vi "NI 5772 (AC) - Digitizer_vDirectDataSend (FPGA) Averaging Try1.vi"() -> ()   [LabVIEW 2020]
doc: "Example Description:\nThis example demonstrates how to enable Time Interleaved Sampling with the NI 5772 adapter module to achieve a sampling rate of 1.6GS/s. This example continuously acquires records of analog input data from the NI 5772 adapter module. It allows you to select an AI channel, trigger type, and record size. This VI must be compiled before it is run. \n\nRunning the VI:\nThis VI must be run from the NI 5772 - Getting Started (Host).vi. Refer to the host VI documentation for steps regarding running and configuring the FPGA VI. \n\nExecution Steps:\nRefer to the Block Diagram of this VI for execution comments."
uses:
  Controls/AI Trigger Type.ctl
  Controls/Aquire State.ctl
  <vilib>/Platform/TimedLoop/XDataNode/timing_clust.ctl
  <vilib>/Platform/TimedLoop/XDataNode/nitl_modes.ctl
  <vilib>/Platform/TimedLoop/XDataNode/wakeup.ctl
  Controls/DigitizerState.ctl
  <vilib>/rvi/Emulation/niFpgaGetClockAttributes.vi
  <vilib>/rvi/Emulation/niFpgaSctlEmulationGetInTimedLoop.vi
  <vilib>/rvi/Emulation/niFpgaEmulationReportErrorSimple.vi
  <vilib>/rvi/eio/common/nirviEmuTemplateMethod_errors.vi
  <vilib>/rvi/Emulation/niFpgaCriticalErrorInLSC.vi
  <vilib>/rvi/Emulation/niFpgaProcessEmulError.vi
  <vilib>/rvi/Emulation/niFpgaEmulationIsFPGAContextNoSignature.vi
  <vilib>/rvi/errors/niFpgaSetErrorForExecOnDevCompSimple.vi
  <vilib>/rvi/eio/common/nirviEmuReportErrorAndStop.vi
  <vilib>/rvi/DataTransferAndStorage/Container/Common/niFpgaContainerGetUniqueNameForEmu.vi
  <vilib>/rvi/FIFO/Fifo_Resource/nirvififoEmulationSetSize.vi
  <vilib>/rvi/FIFO/Fifo_Resource/nirviFifoEmulationQueueMgr.vi
  <instcachedir>/0/nirviFifoEmulationQueueMgr_E5CAEC123FF24DC58D834DCA3CDAA9B5.lvgen/nirviFifoEmulationQueueMgr_E5CAEC123FF24DC58D834DCA3CDAA9B5_004.vi
  <vilib>/Utility/error.llb/Clear Errors.vi
  <vilib>/rvi/FIFO/Fifo_Resource/nirvififoEmulationCreateLock.vi
  <vilib>/rvi/FIFO/Fifo_Resource/nirvififoEmulationObtainLock.vi
  <vilib>/rvi/FIFO/Fifo_Resource/nirvififoEmulationReleaseLock.vi
  <vilib>/rvi/occurrence/nirviWaitOnOccurrenceBase.vi
  <vilib>/rvi/errors/nirviReportUnexpectedCaseInternalError.vi
  <vilib>/rvi/errors/nirviReportUnexpectedCaseInternalError (U32).vi
  <instcachedir>/0/nirviFifoEmulationQueueMgr_E5CAEC123FF24DC58D834DCA3CDAA9B5.lvgen/nirviFifoEmulationQueueMgr_E5CAEC123FF24DC58D834DCA3CDAA9B5_009.vi
  <vilib>/rvi/FIFO/Fifo_Resource/nirvififoEmulationDetermineInputValidOut.vi
  <instcachedir>/0/nirviFifoEmulationQueueMgr_E5CAEC123FF24DC58D834DCA3CDAA9B5.lvgen/nirviFifoEmulationQueueMgr_E5CAEC123FF24DC58D834DCA3CDAA9B5_000.vi
  <vilib>/rvi/interface/RandomDataEmulation/niFpgaRandomDataHandleErrors.vi
  <instrlib>/_niInstr/Basic Elements/v1/FPGA/Private/Count Up U64.vi
  <vilib>/eio/EIONode/EIONode.xnode
  <vilib>/rvi/DataTransferAndStorage/Container/XNode/niFpgaContainer.xnode
  <vilib>/rvi/FIFO/Fifo_Resource/nirvififoEmulationRead.vi
  <vilib>/Platform/TimedLoop/XDataNode/XDataNode.xnode
  <vilib>/rvi/FIFO/Fifo_Resource/nirvififoEmulationGetNumberOfElementsToRead.vi
  <vilib>/rvi/FIFO/Fifo_Resource/nirvififoEmulationWrite.vi
  <vilib>/rvi/interface/RandomDataEmulation/nirviRandomDataFpgaReadWriteTemplate.vi
  <vilib>/Platform/TimedLoop/XDataNode/XDNodeRunTimeDep.lvlib
  <instrlib>/_niInstr/Basic Elements/v1/FPGA/niInstr Basic Elements v1 FPGA.lvlib
  <vilib>/rvi/Memory/Memory_Emulation/nirvimemoryFastEmulation.vi
  <vilib>/rvi/Memory/Memory_Emulation/nirvimemoryEmulation.vi
panel:
  out "DMA FIFO Overflow? 3":bool caption="FIFO Overflow?"
  out "DMA FIFO Overflow? 2":bool caption="FIFO Overflow?"
  out "WaitForWave\nCompletion":u16
  in  "Wave Sampling Rate":sgl
  in  "WaveSampleCount":sgl format="%#_13g"
  in  "Delay (us)":sgl
  in  "AvgCount_powerOf2":i16=1
  out "DMA FIFO Overflow?":bool caption="FIFO Overflow?"
  out "Removed\nElement":u64
  out "AvgCount":u16=1
  in  "vi/nGenTrig":bool
  in  "TrigIn Simulate":bool
  out "Trig Count":u64
  in  "Clear Count":bool
  out "Delay after Trig [cycles]":u16
  out "TS FIFO In Overflow?":bool caption="FIFO Overflow?"
  in  "Samples Per Trigger":u16=512 min=1 step=1
  in  "Arm Trigger":bool
  in  "User Command Commit":bool
  in  "User Command":u8
  out "User Command Idle":bool
  out "User Command Status":u8
  in  "User Data 0":u16
  in  "User Data 1":u8
  out "PLL Locked":bool
  out "User Error":bool
  out "Configured?":bool
  in  "Trigger Level":i16
  in  "Trigger Type":T1
  # "Resource Configuration"
  # "Analog Input"
  # "Clock Configuration"
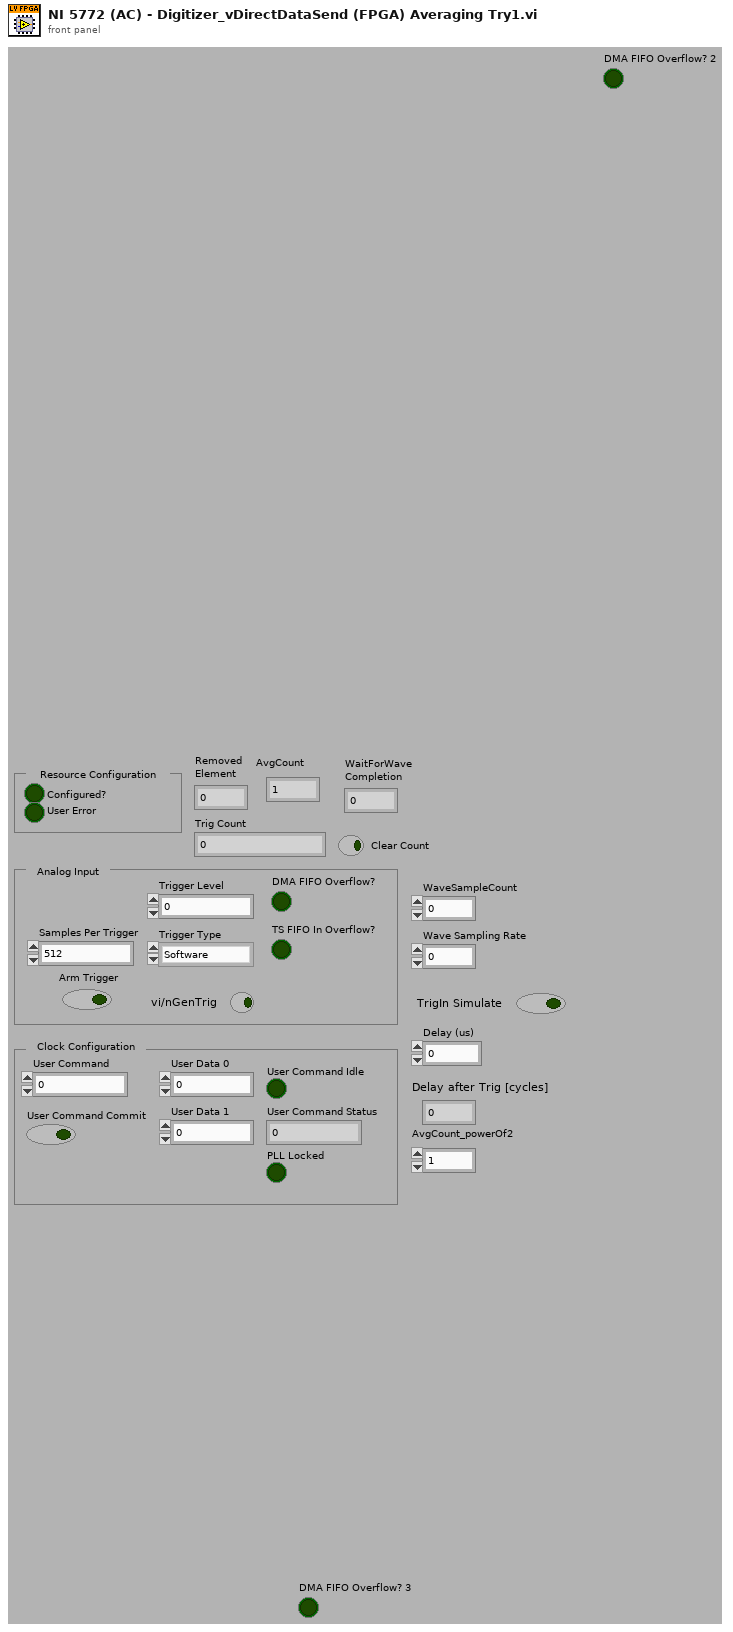
[diagram p1: front panel]
types:
  T1 = typedef "AI Trigger Type.ctl" = enum8{"Software", "Data Edge"}
  T2 = typedef "DigitizerState.ctl" = enum16{"Init", "Build/Clear Accumulator", "GetData", "AverageCountCheck", "SendtoHost"}
  T3 = typedef "Aquire State.ctl" = enum8{"Idle", "Wait for Trigger", "AlignWave", "Hold Aquire", "Acquire", "WaitForWaveCompletion", "CheckAvg"}
  T4 = typedef "XDNodeRunTimeDep.lvlib/timing_clust.ctl" = cluster{"Expected End [f-1]":u64, "Actual End [f-1]":u64, "Finished Late? [f-1]":bool, "Expected End [i-1]":u64, "Actual End [i-1]":u64, "Finished Late? [i-1]":bool, "Expected Start [i]":u64, "Actual Start [i]":u64, "Expected Start [f]":u64, "Actual Start [f]":u64, "Source Name":string, "Structure Name":string, "Period":i64, "Deadline":i64, "Offset":i64, "Start":i64, "Priority":i32, "Timeout":i32, "Mode":T5, "Wakeup Reason":T6, "Error":errorcluster, "Source Type":string, "Secondary Source Type":string, "Global End Time":u64, "Global Start Time":u64, "Frame Duration":u64, "Iteration Duration":u64, "Assigned CPU":i32, "I/O Scan Engine Mode":u32}
  T5 = typedef "XDNodeRunTimeDep.lvlib/nitl_modes.ctl" = enum32{"No Change", "Process missed periods, maintain original phase", "Discard missed periods, maintain original phase", "Process missed periods, ignore original phase", "Discard missed periods, ignore original phase"}
  T6 = typedef "XDNodeRunTimeDep.lvlib/wakeup.ctl" = enum32{"Normal", "Aborted", "Asynchronous wakeup", "Timing source error", "Timed loop error", "Timeout"}
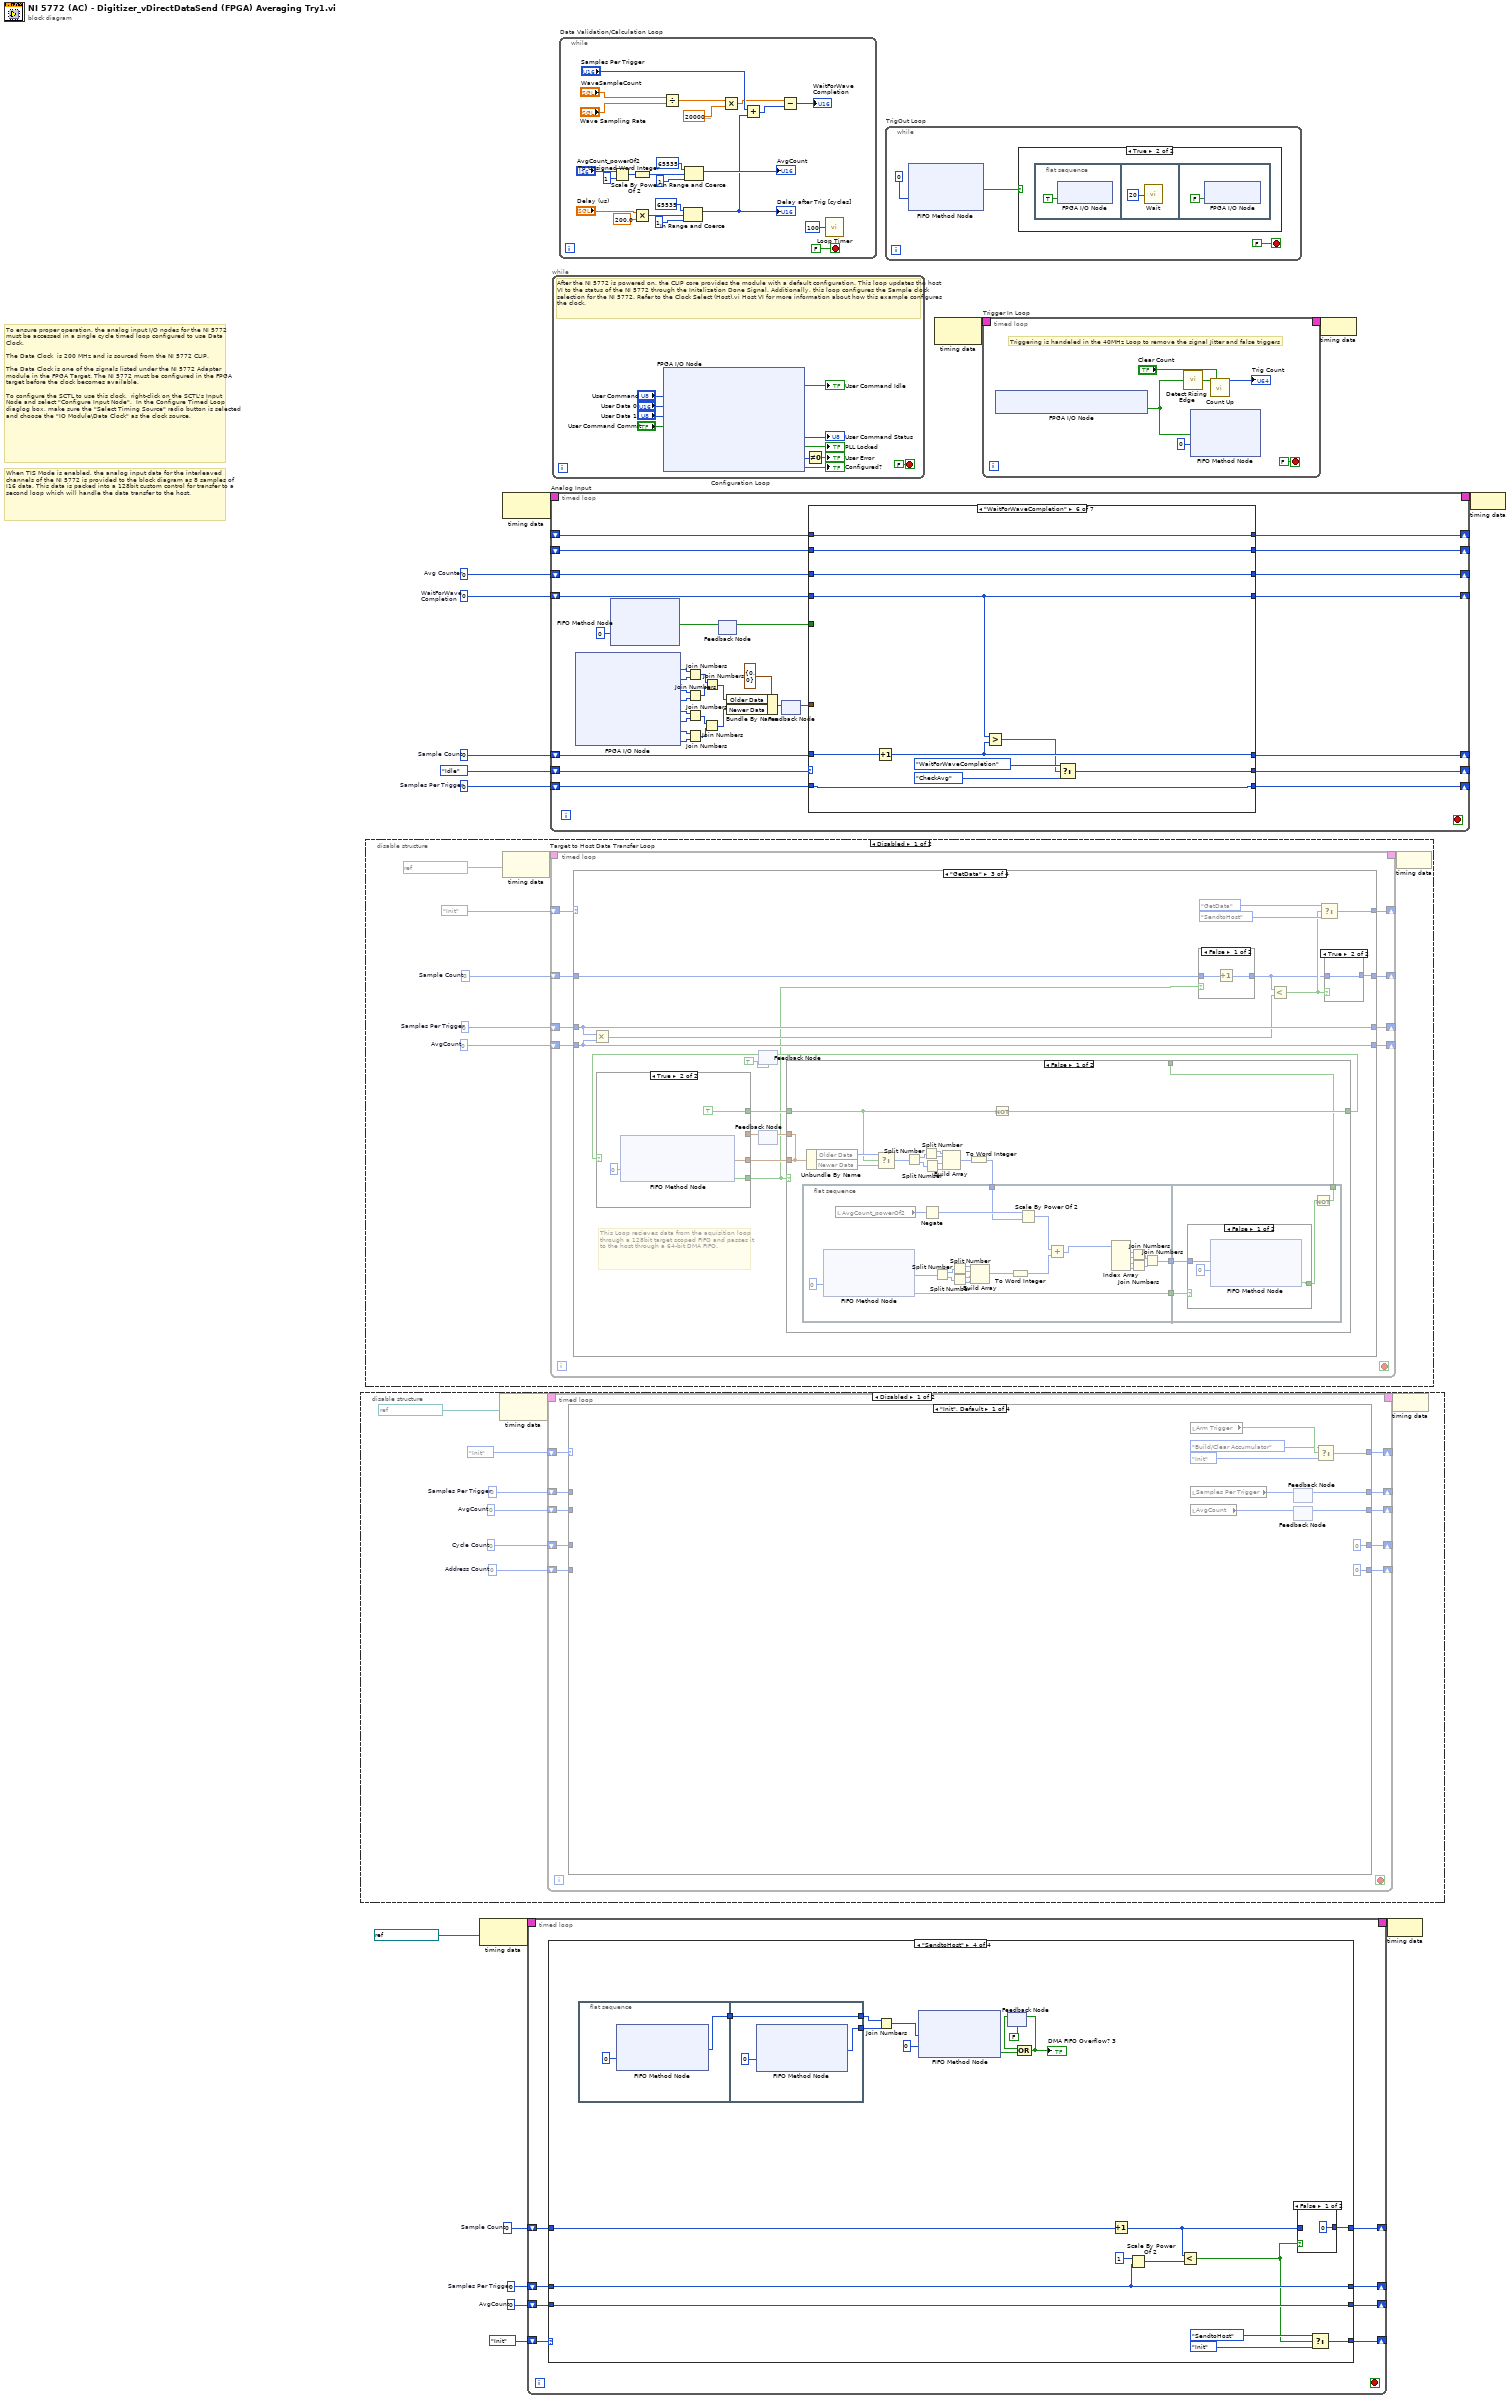
[diagram p0: block diagram]
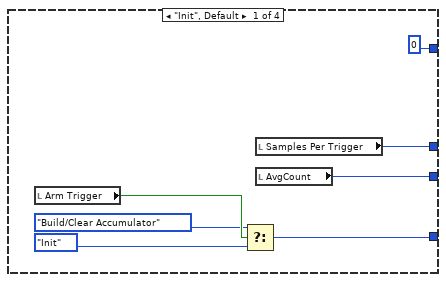
[diagram p2: hidden frame]
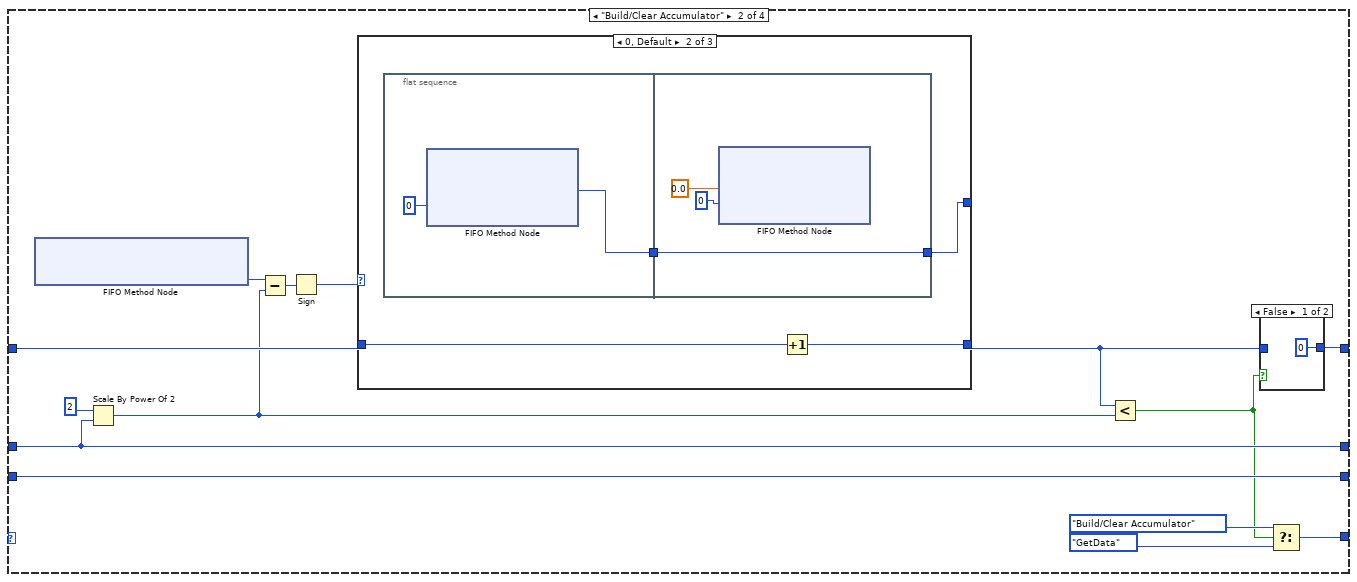
[diagram p3: hidden frame]
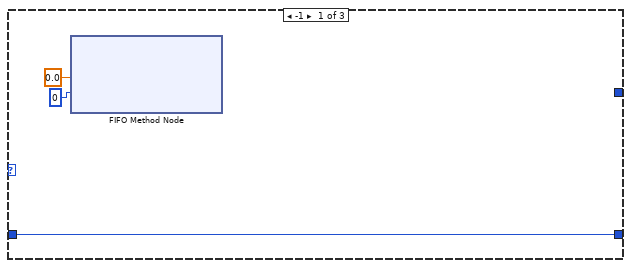
[diagram p5: hidden frame]
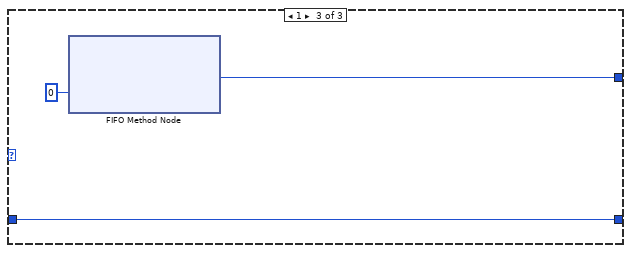
[diagram p6: hidden frame]
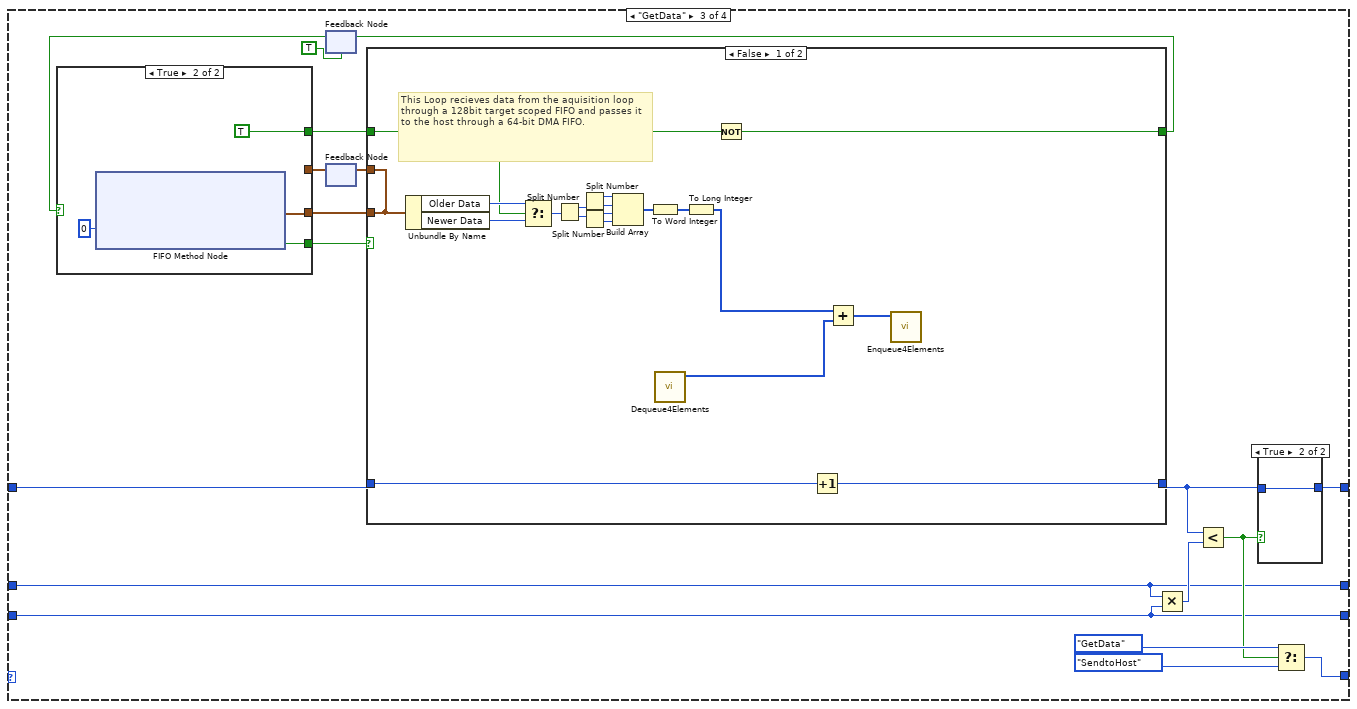
[diagram p7: hidden frame]
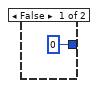
[diagram p8: hidden frame]
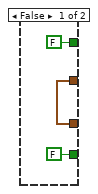
[diagram p9: hidden frame]
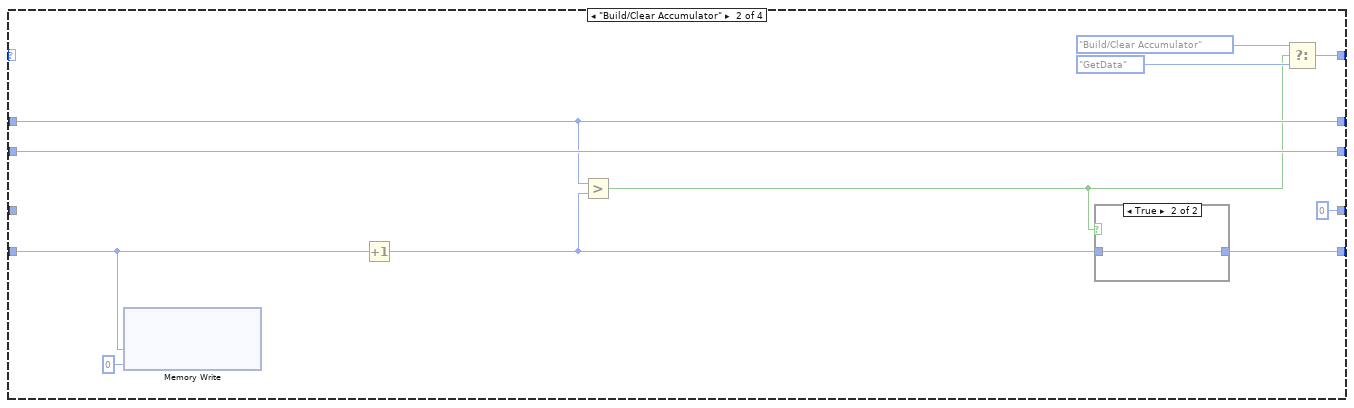
[diagram p12: hidden frame]
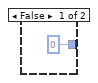
[diagram p13: hidden frame]
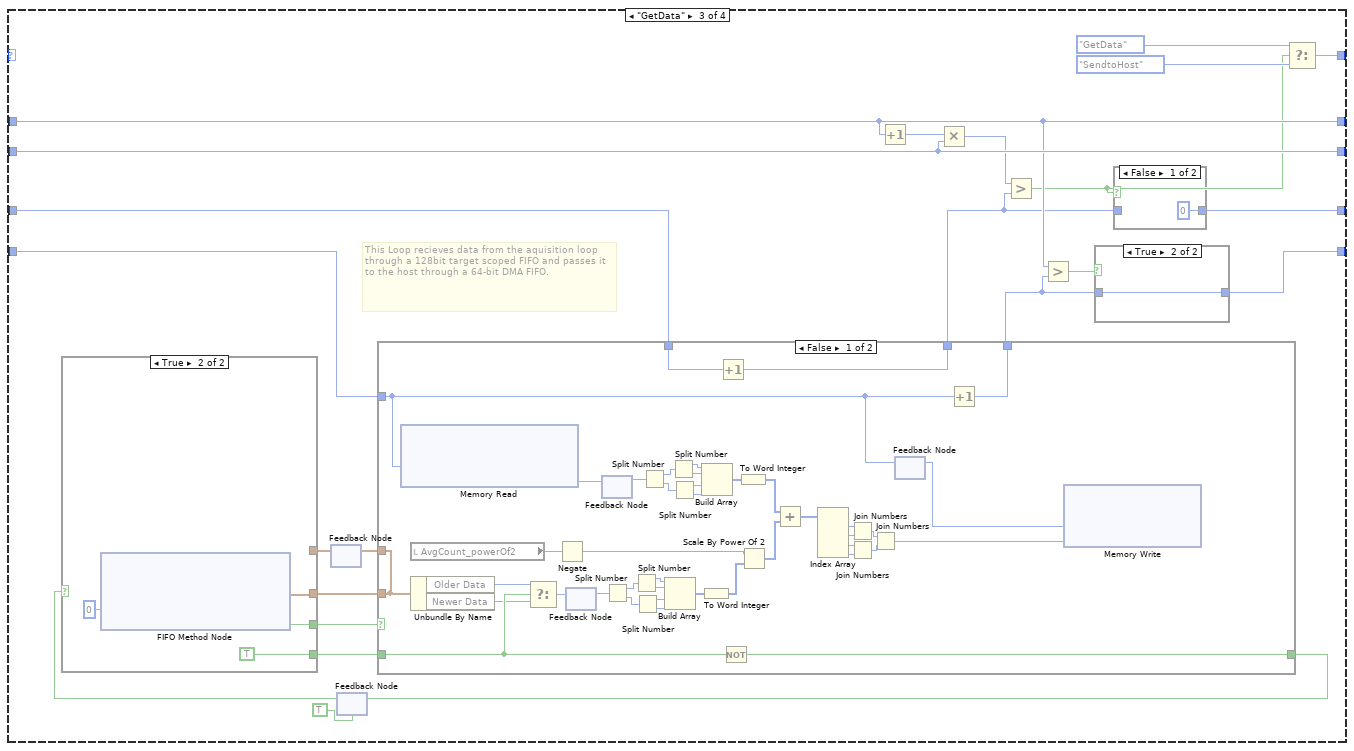
[diagram p14: hidden frame]
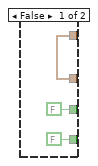
[diagram p16: hidden frame]
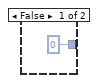
[diagram p18: hidden frame]
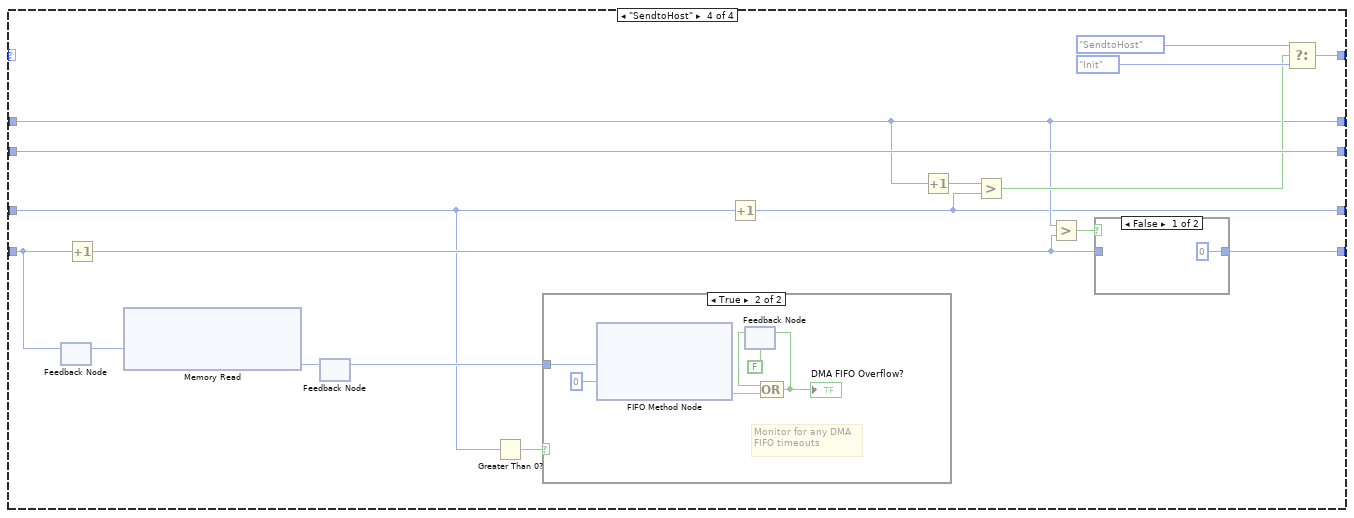
[diagram p19: hidden frame]
diagram:
  w1 = u16 0  # Sample Count
  w2 = u16 0  # AvgCount
  w3 = u16 0  # Samples Per Trigger
  w8 = u16 0  # WaitForWave Completion
  w9 = u16 0  # Avg Counter
  w12 = u16 0  # Samples Per Trigger
  w13 = u16 0  # Sample Count
  # "When TIS Mode is enabled, the analog input data for the interleaved channels of the NI 5772 is provided to the block diagram as 8 samples of I16 data. This data is packed into a 128bit custom control for transfer to a second loop which will handle the data transfer to the host."
  # "To ensure proper operation, the analog input I/O nodes for the NI 5772 must be accessed in a single cycle timed loop configured to use Data Clock. \n\nThe Data Clock  is 200 MHz and is sourced from the NI 5772 CLIP.\n\nThe Data Clock is one of the signals listed under the NI 5772 Adapter module in the FPGA Target. The NI 5772 must be configured in the FPGA target before the clock becomes available. \n\nTo configure the SCTL to use this clock,  right-click on the SCTL's Input Node and select \"Configure Input Node\".  In the Configure Timed Loop diaglog box, make sure the \"Select Timing Source\" radio button is selected and choose the \"IO Module\\Data Clock\" as the clock source."
  n1 = disable-structure shown="Disabled" {
    frame Disabled {
      w17 = u32 0  # Cycle Count
      w18 = u32 0  # Address Count
      w19 = u16 0  # AvgCount
      w20 = u16 0  # Samples Per Trigger
      n2 = node-c288(refnum<k21> "100 MHz Clock" ("Source Name")) -> (w24:T4)
      n3 = timed-loop {
        timing: w24 -> [_]
        timing-out: [_] -> w23
        shift-right: [w33] -> _
        shift-left: DigitizerState."Init" -> [w34]
        shift-right: [w32] -> _
        shift-left: w20 -> [w30]
        shift-right: [w31] -> _
        shift-left: w19 -> [w29]
        shift-right: [w27] -> _
        shift-left: w18 -> [w28]
        shift-right: [w25] -> _
        shift-left: w17 -> [w26]
        stop <- _ stop-if-true
        n4 = case shown="\"Init\", Default" w34 {
          tunnel: [w39 w49 w78 w150] -> w33
          tunnel: [w38 w52 w62 w140] -> w32
          tunnel: [w37 w53 w68 w153] -> w31
          tunnel: w30 -> [_ w52 w62 w140]
          tunnel: w29 -> [_ w53 w68 w153]
          tunnel: w28 -> [_ w55 w65 w142]
          tunnel: [u32 0 w46 w77 w148] -> w27
          tunnel: w26 -> [_ _ w61 w137]
          tunnel: [u32 0 ("Cycle Count") u32 0 ("Cycle Count") w58 w138] -> w25
          frame "Init", Default {
            n5 = local read "Arm Trigger"() -> (w44:bool)
            n6 = local read "Samples Per Trigger"() -> (w40:u16)
            n7 = local read "AvgCount"() -> (w41:u16)
            n8 = feedback #1() -> (w38:u16)  [unwired: 1 in]
            n9 = feedback-in #1(w40) -> ()
            n10 = feedback #2() -> (w37:u16)  [unwired: 1 in]
            n11 = feedback-in #2(w41) -> ()
            n12 = Select(t=DigitizerState."Build/Clear Accumulator", s=w44, f=DigitizerState."Init") -> (s? t:f=w39:T2)
          }
          frame "Build/Clear Accumulator" {
            n13 = xnode ("Memory Write")("Address"=w55, "Data"=u64 0) -> ()  [unwired: 1 in, 1 out]
            n14 = Increment(x=w55) -> (x+1=w47:u32)
            n15 = Greater?(x=w52, y=w47) -> (0:w48:bool)
            n16 = case shown="True" w48 {
              tunnel: w47 -> [_ w57]
              tunnel: [u32 0 w57] -> w46
              frame False {
              }
              frame True {
              }
            }
            n17 = Select(t=DigitizerState."Build/Clear Accumulator", s=w48, f=DigitizerState."GetData") -> (s? t:f=w49:T2)
          }
          frame "GetData" {
            # "This Loop recieves data from the aquisition loop through a 128bit target scoped FIFO and passes it to the host through a 64-bit DMA FIFO."
            n18 = feedback #3() -> (w72:cluster{"Older Data":u64, "Newer Data":u64})  [unwired: 1 in]
            n19 = feedback #4(TRUE ("Timed Out?")) -> (w71:bool)
            n20 = case shown="True" w71 {
              tunnel: [w83 w86] -> w74
              tunnel: [FALSE ("Timed Out?") w87] -> w76
              tunnel: [FALSE ("Timed Out?") TRUE ("Timed Out?")] -> w75
              tunnel: w72 -> [w83 _]
              frame False {
              }
              frame True {
                n21 = xnode ("FIFO Method Node")("Timeout"=0) -> ("Element"=w86:cluster{"Older Data":u64, "Newer Data":u64}, "Timed Out?"=w87:bool)  [unwired: 1 in, 1 out]
              }
            }
            n22 = case shown="False" w76 {
              tunnel: [w128 w134] -> w70
              tunnel: w75 -> [w129 w134]
              tunnel: w74 -> [w127 w133]
              tunnel: [w127 w133] -> w73
              tunnel: w65 -> [w104 w132]
              tunnel: [w117 w132] -> w64
              tunnel: w61 -> [w93 w131]
              tunnel: [w92 w131] -> w59
              frame False {
                n23 = xnode ("Memory Read")("Address"=w104) -> ("Data"=w95:u64)  [unwired: 1 in, 1 out]
                n24 = local read "AvgCount_powerOf2"() -> (w108:i16)
                n25 = Unbundle By Name(w127) -> ("Older Data"=w130:u64, "Newer Data"=w126:u64)
                n26 = Select(t=w130, s=w129, f=w126) -> (s? t:f=w118:u64)
                n27 = Negate(x=w108) -> (-x=w109:i16)
                n28 = feedback-in #5(w118) -> ()
                n29 = feedback #5() -> (w91:u64)  [unwired: 1 in]
                n30 = feedback-in #6(w95) -> ()
                n31 = feedback #6() -> (w94:u64)  [unwired: 1 in]
                n32 = Split Number(x=w91) -> (hi(x)=w120:u32, lo(x)=w121:u32)
                n33 = Split Number(x=w120) -> (hi(x)=w122:u16, lo(x)=w123:u16)
                n34 = Split Number(x=w121) -> (hi(x)=w124:u16, lo(x)=w125:u16)
                n35 = Split Number(x=w94) -> (hi(x)=w116:u32, lo(x)=w115:u32)
                n36 = Build Array(w122, w123, w124, w125) -> (w119:u16[])
                n37 = Split Number(x=w116) -> (hi(x)=w114:u16, lo(x)=w113:u16)
                n38 = Split Number(x=w115) -> (hi(x)=w112:u16, lo(x)=w111:u16)
                n39 = To Word Integer(number=w119) -> (16bit integer=w107:i16[])
                n40 = Build Array(w114, w113, w112, w111) -> (w110:u16[])
                n41 = Increment(x=w93) -> (x+1=w92:u32)
                n42 = Not(x=w129) -> (.not. x?=w128:bool)
                n43 = To Word Integer(number=w110) -> (16bit integer=w105:i16[])
                n44 = Scale By Power Of 2(n=w109, x=w107) -> (x*2^n=w106:i16[])
                n45 = Add(x=w105, y=w106) -> (x+y=w97:i16[])
                n46 = Index Array(array=w97) -> (element #1=w100:i16, element #2=w101:i16, element #3=w102:i16, element #4=w103:i16)  [unwired: 4 in]
                n47 = Join Numbers(hi=w100, lo=w101) -> ((hi.lo)=w98:u32)
                n48 = Join Numbers(hi=w102, lo=w103) -> ((hi.lo)=w99:u32)
                n49 = Join Numbers(hi=w98, lo=w99) -> ((hi.lo)=w96:u64)
                n50 = feedback-in #7(w104) -> ()
                n51 = feedback #7() -> (w90:u32)  [unwired: 1 in]
                n52 = Increment(x=w104) -> (x+1=w117:u32)
                n53 = xnode ("Memory Write")("Address"=w90, "Data"=w96) -> ()  [unwired: 1 in, 1 out]
              }
              frame True {
              }
            }
            n54 = feedback-in #3(w73) -> ()
            n55 = feedback-in #4(w70) -> ()
            n56 = Increment(x=w62) -> (x+1=w63:u16)
            n57 = Multiply(x=w63, y=w68) -> (x*y=w67:u16)
            n58 = Greater?(x=w67, y=w59) -> (0:w60:bool)
            n59 = Greater?(x=w62, y=w64) -> (0:w66:bool)
            n60 = case shown="True" w66 {
              tunnel: w64 -> [_ w136]
              tunnel: [u32 0 w136] -> w77
              frame False {
              }
              frame True {
              }
            }
            n61 = case shown="False" w60 {
              tunnel: w59 -> [_ w82]
              tunnel: [u32 0 ("Cycle Count") w82] -> w58
              frame False {
              }
              frame True {
              }
            }
            n62 = Select(t=DigitizerState."GetData", s=w60, f=DigitizerState."SendtoHost") -> (s? t:f=w78:T2)
          }
          frame "SendtoHost" {
            n63 = feedback-in #8(w142) -> ()
            n64 = feedback #8() -> (w144:u32)  [unwired: 1 in]
            n65 = Increment(x=w142) -> (x+1=w139:u32)
            n66 = xnode ("Memory Read")("Address"=w144) -> ("Data"=w147:u64)  [unwired: 1 in, 1 out]
            n67 = feedback-in #9(w147) -> ()
            n68 = feedback #9() -> (w146:u64)  [unwired: 1 in]
            n69 = Greater Than 0?(x=w137) -> (x > 0?=w143:bool)
            n70 = case shown="True" w143 {
              tunnel: w146 -> [_ w154]
              frame False {
              }
              frame True {
                # "Monitor for any DMA FIFO timeouts"
                n71 = xnode ("FIFO Method Node")("Element"=w154, "Timeout"=0) -> ("Timed Out?"=w158:bool)  [unwired: 1 in, 1 out]
                n72 = feedback #10(FALSE) -> (w157:bool)
                n73 = Compound Arithmetic op=OR(w157, w158) -> (w159:bool)
                "DMA FIFO Overflow?" <- w159
                n74 = feedback-in #10(w159) -> ()
              }
            }
            n75 = Increment(x=w137) -> (x+1=w138:u32)
            n76 = Increment(x=w140) -> (x+1=w145:u16)
            n77 = Greater?(x=w145, y=w138) -> (0:w149:bool)
            n78 = Greater?(x=w140, y=w139) -> (0:w141:bool)
            n79 = case shown="False" w141 {
              tunnel: w139 -> [_ w161]
              tunnel: [u32 0 w161] -> w148
              frame False {
              }
              frame True {
              }
            }
            n80 = Select(t=DigitizerState."SendtoHost", s=w149, f=DigitizerState."Init") -> (s? t:f=w150:T2)
          }
        }
      }
      n81 = node-c288(w23) -> ()
    }
    frame Enabled {
    }
  }
  n82 = disable-structure shown="Disabled" {
    frame Disabled {
      w168 = u16 0  # Sample Count
      w169 = u16 0  # Samples Per Trigger
      w170 = u16 0  # AvgCount
      n83 = node-c288(refnum<k21> "100 MHz Clock" ("Source Name")) -> (w174:T4)
      n84 = timed-loop "Target to Host Data Transfer Loop" {
        timing: w174 -> [_]
        timing-out: [_] -> w173
        shift-right: [w177] -> _
        shift-left: DigitizerState."Init" -> [w182]
        shift-right: [w181] -> _
        shift-left: w169 -> [w180]
        shift-right: [w179] -> _
        shift-left: w170 -> [w178]
        shift-right: [w175] -> _
        shift-left: w168 -> [w176]
        stop <- _ stop-if-true
        n85 = case shown="\"GetData\"" w182 {
          tunnel: [w190 w195 w243 w317] -> w181
          tunnel: w180 -> [_ w195 w243 w317]
          tunnel: [w188 w196 w242 w324] -> w179
          tunnel: w178 -> [_ w196 w242 w324]
          tunnel: [w184 w203 w237 w320] -> w177
          tunnel: w176 -> [_ w198 w236 w318]
          tunnel: [u16 0 ("Sample Count") w192 w235 w315] -> w175
          frame "Init", Default {
            n86 = local read "Arm Trigger"() -> (w185:bool)
            n87 = local read "Samples Per Trigger"() -> (w191:u16)
            n88 = local read "AvgCount"() -> (w189:u16)
            n89 = feedback #11() -> (w190:u16)  [unwired: 1 in]
            n90 = feedback-in #11(w191) -> ()
            n91 = feedback #12() -> (w188:u16)  [unwired: 1 in]
            n92 = feedback-in #12(w189) -> ()
            n93 = Select(t=DigitizerState."Build/Clear Accumulator", s=w185, f=DigitizerState."Init") -> (s? t:f=w184:T2)
          }
          frame "Build/Clear Accumulator" {
            n94 = xnode ("FIFO Method Node")() -> ("Number of Elements to Read"=w207:u32)  [unwired: 1 in, 1 out]
            n95 = Subtract(x=w207, y=w195) -> (x-y=w206:i8)
            n96 = Sign(1:w206) -> (0:w205:i8)
            n97 = case shown="-1" w205 {
              tunnel: [_ w220 w231] -> w204
              tunnel: [w214 w218 w230] -> w200
              tunnel: [FALSE TRUE FALSE] -> w199
              frame -1 {
                n98 = xnode ("FIFO Method Node")("Element"=u64 0, "Timeout"=0) -> ("Timed Out?"=w214:bool)  [unwired: 1 in, 1 out]
              }
              frame 0, Default {
                n99 = flat-sequence {
                  tunnel: [w222] -> w220
                  tunnel: [w221] -> w219
                  tunnel: w219 -> [w226]
                  tunnel: [w224] -> w218
                  frame #0 {
                    n100 = xnode ("FIFO Method Node")("Timeout"=0) -> ("Element"=w222:i32, "Timed Out?"=w221:bool)  [unwired: 1 in, 1 out]
                  }
                  frame #1 {
                    n101 = xnode ("FIFO Method Node")("Element"=u64 0 ("y"), "Timeout"=0) -> ("Timed Out?"=w225:bool)  [unwired: 1 in, 1 out]
                    n102 = Compound Arithmetic op=OR(w226, w225) -> (w224:bool)
                  }
                }
              }
              frame 1 {
                n103 = xnode ("FIFO Method Node")("Timeout"=0) -> ("Element"=w231:i32, "Timed Out?"=w230:bool)  [unwired: 1 in, 1 out]
              }
            }
            "Removed\nElement" <- w204
            n104 = Compound Arithmetic op=AND(invert w200, w199) -> (w197:bool)
            n105 = case shown="True" w197 {
              tunnel: w198 -> [w210 w212]
              tunnel: [w210 w211] -> w193
              frame False {
              }
              frame True {
                n106 = Increment(x=w212) -> (x+1=w211:u16)
              }
            }
            n107 = Less?(x=w193, y=w195) -> (x < y?=w194:bool)
            n108 = Select(t=DigitizerState."Build/Clear Accumulator", s=w194, f=DigitizerState."GetData") -> (s? t:f=w203:T2)
            n109 = case shown="True" w194 {
              tunnel: [u16 0 ("Sample Count") w209] -> w192
              tunnel: w193 -> [_ w209]
              frame False {
              }
              frame True {
              }
            }
          }
          frame "GetData" {
            # "This Loop recieves data from the aquisition loop through a 128bit target scoped FIFO and passes it to the host through a 64-bit DMA FIFO."
            n110 = Multiply(x=w243, y=w242) -> (x*y=w234:u16)
            n111 = feedback #13(TRUE ("Timed Out?")) -> (w248:bool)
            n112 = feedback #14() -> (w247:cluster{"Older Data":u64, "Newer Data":u64})  [unwired: 1 in]
            n113 = case shown="True" w248 {
              tunnel: [w256 w259] -> w245
              tunnel: [FALSE ("Timed Out?") w260] -> w233
              tunnel: [FALSE ("Timed Out?") TRUE ("Timed Out?")] -> w244
              tunnel: w247 -> [w256 _]
              frame False {
              }
              frame True {
                n114 = xnode ("FIFO Method Node")("Timeout"=0) -> ("Element"=w259:cluster{"Older Data":u64, "Newer Data":u64}, "Timed Out?"=w260:bool)  [unwired: 1 in, 1 out]
              }
            }
            n115 = case shown="False" w233 {
              tunnel: [w277 w313] -> w249
              tunnel: w244 -> [w278 w313]
              tunnel: w245 -> [w276 w312]
              tunnel: [w276 w312] -> w246
              tunnel: [w264 FALSE ("increment")] -> _
              frame False {
                n116 = flat-sequence {
                  tunnel: [w280] -> w268
                  tunnel: [w291] -> w266
                  tunnel: w263 -> [w287]
                  tunnel: w268 -> [w306]
                  tunnel: [w303] -> w264
                  tunnel: w266 -> [w305]
                  frame #0 {
                    n117 = xnode ("FIFO Method Node")("Timeout"=0) -> ("Element"=w290:i32, "Timed Out?"=w291:bool)  [unwired: 1 in, 1 out]
                    n118 = local read "AvgCount_powerOf2"() -> (w289:i16)
                    n119 = Negate(x=w289) -> (-x=w288:i16)
                    n120 = Split Number(x=w290) -> (hi(x)=w296:u16, lo(x)=w297:u16)
                    n121 = Split Number(x=w296) -> (hi(x)=w298:u8, lo(x)=w299:u8)
                    n122 = Split Number(x=w297) -> (hi(x)=w300:u8, lo(x)=w301:u8)
                    n123 = Build Array(w298, w299, w300, w301) -> (w302:u8[])
                    n124 = To Word Integer(number=w302) -> (16bit integer=w294:i16[])
                    n125 = Scale By Power Of 2(n=w288, x=w287) -> (x*2^n=w286:i16[])
                    n126 = Add(x=w286, y=w294) -> (x+y=w285:i16[])
                    n127 = Index Array(array=w285) -> (element #1=w284:i16, element #2=w283:i16, element #3=w282:i16, element #4=w281:i16)  [unwired: 4 in]
                    n128 = Join Numbers(hi=w284, lo=w283) -> ((hi.lo)=w293:u32)
                    n129 = Join Numbers(hi=w282, lo=w281) -> ((hi.lo)=w292:u32)
                    n130 = Join Numbers(hi=w293, lo=w292) -> ((hi.lo)=w280:u64)
                  }
                  frame #1 {
                    n131 = case shown="False" w305 {
                      tunnel: w306 -> [w308 _]
                      tunnel: [w307 TRUE ("Timed Out?")] -> w304
                      frame False {
                        n132 = xnode ("FIFO Method Node")("Element"=w308, "Timeout"=0) -> ("Timed Out?"=w307:bool)  [unwired: 1 in, 1 out]
                      }
                      frame True {
                      }
                    }
                    n133 = Not(x=w304) -> (.not. x?=w303:bool)
                  }
                }
                n134 = Unbundle By Name(w276) -> ("Older Data"=w279:u64, "Newer Data"=w275:u64)
                n135 = Select(t=w279, s=w278, f=w275) -> (s? t:f=w265:u64)
                n136 = Split Number(x=w265) -> (hi(x)=w269:u32, lo(x)=w270:u32)
                n137 = Split Number(x=w269) -> (hi(x)=w271:u16, lo(x)=w272:u16)
                n138 = Split Number(x=w270) -> (hi(x)=w273:u16, lo(x)=w274:u16)
                n139 = Build Array(w271, w272, w273, w274) -> (w267:u16[])
                n140 = To Word Integer(number=w267) -> (16bit integer=w263:i16[])
                n141 = Not(x=w278) -> (.not. x?=w277:bool)
              }
              frame True {
              }
            }
            n142 = feedback-in #13(w249) -> ()
            n143 = feedback-in #14(w246) -> ()
            n144 = case shown="False" w233 {
              tunnel: w236 -> [w254 w255]
              tunnel: [w253 w255] -> w238
              frame False {
                n145 = Increment(x=w254) -> (x+1=w253:u16)
              }
              frame True {
              }
            }
            n146 = Less?(x=w238, y=w234) -> (x < y?=w239:bool)
            n147 = Select(t=DigitizerState."GetData", s=w239, f=DigitizerState."SendtoHost") -> (s? t:f=w237:T2)
            n148 = case shown="True" w239 {
              tunnel: [u16 0 ("Sample Count") w252] -> w235
              tunnel: w238 -> [_ w252]
              frame False {
              }
              frame True {
              }
            }
          }
          frame "SendtoHost" {
            n149 = xnode ("FIFO Method Node")("Timeout"=0) -> ("Element"=w323:i32, "Timed Out?"=w314:bool)  [unwired: 1 in, 1 out]
            n150 = case shown="False" w314 {
              tunnel: w323 -> [w326 _]
              frame False {
                n151 = xnode ("FIFO Method Node")("Element"=w326, "Timeout"=0) -> ("Timed Out?"=w328:bool)  [unwired: 1 in, 1 out]
                n152 = feedback #15(FALSE) -> (w329:bool)
                n153 = Compound Arithmetic op=OR(w329, w328) -> (w327:bool)
                "DMA FIFO Overflow? 2" <- w327
                n154 = feedback-in #15(w327) -> ()
              }
              frame True {
              }
            }
            n155 = Increment(x=w318) -> (x+1=w319:u16)
            n156 = Less?(x=w319, y=w317) -> (x < y?=w316:bool)
            n157 = case shown="False" w316 {
              tunnel: [u16 0 ("Sample Count") w333] -> w315
              tunnel: w319 -> [_ w333]
              frame False {
              }
              frame True {
              }
            }
            n158 = Select(t=DigitizerState."SendtoHost", s=w316, f=DigitizerState."Init") -> (s? t:f=w320:T2)
          }
        }
      }
      n159 = node-c288(w173) -> ()
    }
    frame Enabled {
    }
  }
  n160 = node-c288(refnum<k21> "100 MHz Clock" ("Source Name")) -> (w7:T4)
  n161 = node-c288() -> (w16:T4)  [unwired: 1 in]
  n162 = timed-loop {
    timing: w7 -> [_]
    timing-out: [_] -> w6
    shift-right: [w340] -> _
    shift-left: DigitizerState."Init" -> [w347]
    shift-right: [w345] -> _
    shift-left: w3 -> [w344]
    shift-right: [w346] -> _
    shift-left: w2 -> [w343]
    shift-right: [w341] -> _
    shift-left: w1 -> [w342]
    stop <- _ stop-if-true
    n163 = case shown="\"SendtoHost\"" w347 {
      tunnel: [w354 w366 w386 w453] -> w346
      tunnel: [w353 w367 w387 w452] -> w345
      tunnel: w344 -> [_ w367 w387 w452]
      tunnel: w343 -> [_ w366 w386 w453]
      tunnel: w342 -> [_ w362 w395 w454]
      tunnel: [u16 0 ("Sample Count") w357 w391 w447] -> w341
      tunnel: [w348 w358 w392 w449] -> w340
      frame "Init", Default {
        n164 = local read "Arm Trigger"() -> (w351:bool)
        n165 = Select(t=DigitizerState."Build/Clear Accumulator", s=w351, f=DigitizerState."Init") -> (s? t:f=w348:T2)
        n166 = local read "Samples Per Trigger"() -> (w353:u16)
        n167 = local read "AvgCount"() -> (w354:u16)
      }
      frame "Build/Clear Accumulator" {
        n168 = xnode ("FIFO Method Node")() -> ("Number of Elements to Read"=w364:u32)  [unwired: 1 in, 1 out]
        n169 = Scale By Power Of 2(n=i16 2, x=w367) -> (x*2^n=w361:u16)
        n170 = Subtract(x=w364, y=w361) -> (x-y=w365:i8)
        n171 = Sign(1:w365) -> (0:w363:i8)
        n172 = case shown="0, Default" w363 {
          tunnel: [_ w375 w384] -> _
          tunnel: [w371 w377 w383] -> w356
          tunnel: w362 -> [w371 w376 w383]
          frame -1 {
            n173 = xnode ("FIFO Method Node")("Element"=sgl 0.0, "Timeout"=0) -> ()  [unwired: 1 in, 2 out]
          }
          frame 0, Default {
            n174 = flat-sequence {
              tunnel: [w378] -> w374
              tunnel: [w380] -> w375
              tunnel: w374 -> [w380]
              frame #0 {
                n175 = xnode ("FIFO Method Node")("Timeout"=0) -> ("Element"=w378:i32)  [unwired: 1 in, 2 out]
              }
              frame #1 {
                n176 = xnode ("FIFO Method Node")("Element"=sgl 0.0 ("y"), "Timeout"=0) -> ()  [unwired: 1 in, 2 out]
              }
            }
            n177 = Increment(x=w376) -> (x+1=w377:u16)
          }
          frame 1 {
            n178 = xnode ("FIFO Method Node")("Timeout"=0) -> ("Element"=w384:i32)  [unwired: 1 in, 2 out]
          }
        }
        n179 = Less?(x=w356, y=w361) -> (x < y?=w355:bool)
        n180 = case shown="False" w355 {
          tunnel: [u16 0 ("Sample Count") w370] -> w357
          tunnel: w356 -> [_ w370]
          frame False {
          }
          frame True {
          }
        }
        n181 = Select(t=DigitizerState."Build/Clear Accumulator", s=w355, f=DigitizerState."GetData") -> (s? t:f=w358:T2)
      }
      frame "GetData" {
        n182 = feedback #16(TRUE ("Timed Out?")) -> (w398:bool)
        n183 = feedback #17() -> (w399:cluster{"Older Data":u64, "Newer Data":u64})  [unwired: 1 in]
        n184 = case shown="True" w398 {
          tunnel: [w406 w409] -> w401
          tunnel: [FALSE ("Timed Out?") w410] -> w403
          tunnel: [FALSE ("Timed Out?") TRUE ("Timed Out?")] -> w402
          tunnel: w399 -> [w406 _]
          frame False {
          }
          frame True {
            n185 = xnode ("FIFO Method Node")("Timeout"=0) -> ("Element"=w409:cluster{"Older Data":u64, "Newer Data":u64}, "Timed Out?"=w410:bool)  [unwired: 1 in, 1 out]
          }
        }
        n186 = case shown="False" w403 {
          tunnel: [w429 w434] -> w397
          tunnel: w402 -> [w430 w434]
          tunnel: w401 -> [w428 w433]
          tunnel: [w428 w433] -> w400
          tunnel: w395 -> [w418 w432]
          tunnel: [w417 w432] -> w390
          frame False {
            # "This Loop recieves data from the aquisition loop through a 128bit target scoped FIFO and passes it to the host through a 64-bit DMA FIFO."
            n187 = Unbundle By Name(w428) -> ("Older Data"=w431:u64, "Newer Data"=w427:u64)
            n188 = Select(t=w431, s=w430, f=w427) -> (s? t:f=w424:u64)
            n189 = Split Number(x=w424) -> (hi(x)=w426:u32, lo(x)=w425:u32)
            n190 = Split Number(x=w426) -> (hi(x)=w423:u16, lo(x)=w422:u16)
            n191 = Split Number(x=w425) -> (hi(x)=w421:u16, lo(x)=w420:u16)
            n192 = Build Array(w423, w422, w421, w420) -> (w419:u16[])
            n193 = To Word Integer(number=w419) -> (16bit integer=w416:i16[])
            n194 = call "Dequeue4Elements.vi"() -> ("Data Out"=w414:i32[])  [unwired: 11 in]
            n195 = To Long Integer(number=w416) -> (32bit integer=w413:i32[])
            n196 = Not(x=w430) -> (.not. x?=w429:bool)
            n197 = Increment(x=w418) -> (x+1=w417:u16)
            n198 = Add(x=w413, y=w414) -> (x+y=w415:i32[])
            n199 = call "Enqueue4Elements.vi"("Data In"=w415) -> ()  [unwired: 11 in]
          }
          frame True {
          }
        }
        n200 = feedback-in #16(w397) -> ()
        n201 = feedback-in #17(w400) -> ()
        n202 = Multiply(x=w387, y=w386) -> (x*y=w388:u16)
        n203 = Less?(x=w390, y=w388) -> (x < y?=w389:bool)
        n204 = case shown="True" w389 {
          tunnel: [u16 0 ("Sample Count") w405] -> w391
          tunnel: w390 -> [_ w405]
          frame False {
          }
          frame True {
          }
        }
        n205 = Select(t=DigitizerState."GetData", s=w389, f=DigitizerState."SendtoHost") -> (s? t:f=w392:T2)
      }
      frame "SendtoHost" {
        n206 = flat-sequence {
          tunnel: [w455] -> w438
          tunnel: [w458] -> w437
          tunnel: w438 -> [w458]
          tunnel: [w457] -> w436
          frame #0 {
            n207 = xnode ("FIFO Method Node")("Timeout"=0) -> ("Element"=w455:i32)  [unwired: 1 in, 2 out]
          }
          frame #1 {
            n208 = xnode ("FIFO Method Node")("Timeout"=0) -> ("Element"=w457:i32)  [unwired: 1 in, 2 out]
          }
        }
        n209 = Join Numbers(hi=w437, lo=w436) -> ((hi.lo)=w435:u64)
        n210 = xnode ("FIFO Method Node")("Element"=w435, "Timeout"=0) -> ("Timed Out?"=w443:bool)  [unwired: 1 in, 1 out]
        n211 = feedback #18(FALSE) -> (w442:bool)
        n212 = Compound Arithmetic op=OR(w442, w443) -> (w444:bool)
        "DMA FIFO Overflow? 3" <- w444
        n213 = feedback-in #18(w444) -> ()
        n214 = Increment(x=w454) -> (x+1=w446:u16)
        n215 = Scale By Power Of 2(n=i16 1, x=w452) -> (x*2^n=w448:u16)
        n216 = Less?(x=w446, y=w448) -> (x < y?=w445:bool)
        n217 = case shown="False" w445 {
          tunnel: [u16 0 ("Sample Count") w461] -> w447
          tunnel: w446 -> [_ w461]
          frame False {
          }
          frame True {
          }
        }
        n218 = Select(t=DigitizerState."SendtoHost", s=w445, f=DigitizerState."Init") -> (s? t:f=w449:T2)
      }
    }
  }
  n219 = timed-loop "Analog Input" {
    timing: w16 -> [_]
    timing-out: [_] -> w15
    shift-right: [w496] -> _
    shift-left: Aquire_State."Idle" ("Acquire State") -> [w486]
    shift-right: [w497] -> _
    shift-left: w13 -> [w487]
    shift-right: [w495] -> _
    shift-left: w12 -> [w485]
    shift-right: [w472] -> _
    shift-left: _ -> [w471]
    shift-right: [w470] -> _
    shift-left: _ -> [w469]
    shift-right: [w467] -> _
    shift-left: w9 -> [w468]
    shift-right: [w465] -> _
    shift-left: w8 -> [w464]
    stop <- _ stop-if-true
    n220 = xnode "FPGA I/O Node"() -> ("IO Module\\AI 1 Data N-3"=w478:i16, "IO Module\\AI 0 Data N-3"=w477:i16, "IO Module\\AI 1 Data N-2"=w476:i16, "IO Module\\AI 0 Data N-2"=w475:i16, "IO Module\\AI 1 Data N-1"=w479:i16, "IO Module\\AI 0 Data N-1"=w480:i16, "IO Module\\AI 1 Data N"=w481:i16, "IO Module\\AI 0 Data N"=w482:i16)  [unwired: 8 in, 8 out]
    n221 = xnode ("FIFO Method Node")("Timeout"=0) -> ("Element"=w473:bool)  [unwired: 1 in, 2 out]
    n222 = Join Numbers(hi=w478, lo=w477) -> ((hi.lo)=w490:u32)
    n223 = Join Numbers(hi=w476, lo=w475) -> ((hi.lo)=w492:u32)
    n224 = Join Numbers(hi=w479, lo=w480) -> ((hi.lo)=w491:u32)
    n225 = Join Numbers(hi=w481, lo=w482) -> ((hi.lo)=w493:u32)
    n226 = Join Numbers(hi=w491, lo=w493) -> ((hi.lo)=w483:u64)
    n227 = Join Numbers(hi=w490, lo=w492) -> ((hi.lo)=w484:u64)
    n228 = feedback-in #19(w473) -> ()
    n229 = feedback #19() -> (w466:bool)  [unwired: 1 in]
    n230 = Bundle By Name(cluster=cluster{"Older Data":u64, "Newer Data":u64} {"Older Data"=0, "Newer Data"=0} ("Element"), "Older Data"=w484, "Newer Data"=w483) -> (w488:cluster{"Older Data":u64, "Newer Data":u64})
    n231 = feedback #20() -> (w494:cluster{"Older Data":u64, "Newer Data":u64})  [unwired: 1 in]
    n232 = feedback-in #20(w488) -> ()
    n233 = case shown="\"WaitForWaveCompletion\"" w486 {
      tunnel: [u16 0 u16 0 w550 w562 w571 w593 u16 0] -> w497
      tunnel: w487 -> [_ _ w550 w561 w586 w595 _]
      tunnel: [w509 w521 w553 w565 w585 w598 w609] -> w496
      tunnel: [w506 w525 w551 w563 w582 w596 w607] -> w495
      tunnel: w485 -> [_ w525 w551 w563 w582 w596 w607]
      tunnel: w494 -> [_ w524 _ _ w581 _ _]
      tunnel: w466 -> [_ w519 _ _ _ _ _]
      tunnel: [w504 w517 w549 w560 w575 w594 w606] -> w472
      tunnel: w471 -> [_ w517 w549 w560 w575 w594 w606]
      tunnel: [w502 w516 w548 w558 w574 w591 w604] -> w470
      tunnel: w469 -> [_ w516 w548 w558 w574 w591 w604]
      tunnel: [u16 0 ("Avg Count") w515 w547 w557 w573 w590 w603] -> w467
      tunnel: w468 -> [_ w515 w547 w557 w573 w590 w605]
      tunnel: [w498 w513 w545 w555 w569 w589 w600] -> w465
      tunnel: w464 -> [_ w513 w545 w555 w569 w589 w600]
      frame "Idle", Default {
        # "This state will wait for the host VI to arm the trigger."
        n234 = feedback-in #21("Arm Trigger") -> ()
        n235 = feedback #21() -> (w507:bool)  [unwired: 1 in]
        n236 = local read "WaitForWave\nCompletion"() -> (w499:u16)
        n237 = Select(t=Aquire_State."Wait for Trigger" ("Acquire State"), s=w507, f=Aquire_State."Idle" ("Acquire State")) -> (s? t:f=w509:T3)
        n238 = local read "Delay after Trig [cycles]"() -> (w505:u16)
        n239 = local read "AvgCount"() -> (w503:u16)
        n240 = local read "Samples Per Trigger"() -> (w500:u16)
        n241 = feedback #22() -> (w504:u16)  [unwired: 1 in]
        n242 = feedback-in #22(w505) -> ()
        n243 = feedback #23() -> (w502:u16)  [unwired: 1 in]
        n244 = feedback-in #23(w503) -> ()
        n245 = feedback #24() -> (w498:u16)  [unwired: 1 in]
        n246 = feedback-in #24(w499) -> ()
        n247 = feedback-in #25(w500) -> ()
        n248 = feedback #25() -> (w506:u16)  [unwired: 1 in]
      }
      frame "Wait for Trigger" {
        # "After the trigger is armed, this state monitors for the specific trigger condition to begin the acquisition."
        n249 = feedback-in #26("Trigger Type") -> ()
        n250 = feedback #26() -> (w518:T1)  [unwired: 1 in]
        n251 = case shown="\"Software\", Default" w518 {
          tunnel: w524 -> [_ w544]
          tunnel: [w535 w536] -> w514
          tunnel: w519 -> [w530 _]
          frame "Software", Default {
            n252 = Compound Arithmetic op=AND(w530, invert "vi/nGenTrig") -> (w534:bool)
            n253 = Compound Arithmetic op=AND("vi/nGenTrig", "TrigIn Simulate") -> (w532:bool)
            n254 = Compound Arithmetic op=OR(w534, w532) -> (w529:bool)
            n255 = call <instrlib>:"Detect Rising Edge.vi"("signal"=w529) -> ("edge detected"=w535:bool)  [unwired: 14 in]
          }
          frame "Data Edge" {
            # "Begins the acquisition after the analog input rises above the trigger level."
            n256 = Unbundle By Name(w544) -> ("Older Data"=w542:u64, "Newer Data"=w540:u64)
            n257 = feedback-in #27("Trigger Level") -> ()
            n258 = feedback #27() -> (w538:i16)  [unwired: 1 in]
            n259 = feedback-in #28(w542) -> ()
            n260 = feedback #28() -> (w537:u64)  [unwired: 1 in]
            n261 = feedback-in #29(w540) -> ()
            n262 = feedback #29() -> (w539:u64)  [unwired: 1 in]
            n263 = call "Data Edge Trigger 8 Samples.vi"("Trigger Level"=w538, "Newer Data In"=w539, "Older Data In"=w537) -> ("Trigger"=w543:bool)  [unwired: 8 in]
            n264 = feedback-in #30(w543) -> ()
            n265 = feedback #30() -> (w536:bool)  [unwired: 1 in]
          }
        }
        n266 = case shown="True" w514 {
          selector: w514 -> [_ w528]
          frame False {
          }
          frame True {
            n267 = xnode ("FIFO Method Node")("Element"=w528, "Timeout"=0) -> ()  [unwired: 1 in, 2 out]
          }
        }
        n268 = Select(t=Aquire_State."AlignWave" ("Acquire State"), s=w514, f=Aquire_State."Wait for Trigger") -> (s? t:f=w521:T3)
      }
      frame "AlignWave" {
        n269 = xnode "FPGA I/O Node"() -> ("PXI_Trig0"=w546:bool)  [unwired: 1 in, 1 out]
        n270 = Select(t=Aquire_State."Hold Aquire" ("Acquire State"), s=w546, f=Aquire_State."AlignWave" ("Acquire State")) -> (s? t:f=w553:T3)
      }
      frame "Hold Aquire" {
        n271 = Increment(x=w561) -> (x+1=w559:u16)
        n272 = Greater?(x=w560, y=w559) -> (0:w556:bool)
        n273 = Select(t=Aquire_State."Hold Aquire" ("Acquire State"), s=w556, f=Aquire_State."Acquire" ("Acquire State")) -> (s? t:f=w565:T3)
        n274 = case shown="True" w556 {
          tunnel: [u16 0 w568] -> w562
          tunnel: w559 -> [_ w568]
          frame False {
          }
          frame True {
          }
        }
      }
      frame "Acquire" {
        # "Monitor for any  FIFO timeouts"
        # "While in this state, data is pushed into a DMA FIFO until the desired number of samples per record have been acquired."
        n275 = xnode ("FIFO Method Node")("Element"=w581, "Timeout"=0) -> ("Timed Out?"=w576:bool)  [unwired: 1 in, 1 out]
        n276 = Increment(x=w586) -> (x+1=w572:u16)
        n277 = Less?(x=w572, y=w582) -> (x < y?=w570:bool)
        n278 = feedback #31(FALSE) -> (w577:bool)
        n279 = Or(x=w577, y=w576) -> (x .or. y?=w578:bool)
        "TS FIFO In Overflow?" <- w578
        n280 = feedback-in #31(w578) -> ()
        n281 = Select(t=Aquire_State."Acquire" ("Acquire State"), s=w570, f=Aquire_State."WaitForWaveCompletion" ("Acquire State")) -> (s? t:f=w585:T3)
        n282 = case shown="False" w570 {
          tunnel: w572 -> [_ w588]
          tunnel: [u16 0 w588] -> w571
          frame False {
          }
          frame True {
          }
        }
      }
      frame "WaitForWaveCompletion" {
        n283 = Increment(x=w595) -> (x+1=w593:u16)
        n284 = Greater?(x=w589, y=w593) -> (0:w592:bool)
        n285 = Select(t=Aquire_State."WaitForWaveCompletion" ("Acquire State"), s=w592, f=Aquire_State."CheckAvg" ("Acquire State")) -> (s? t:f=w598:T3)
      }
      frame "CheckAvg" {
        n286 = Increment(x=w605) -> (x+1=w603:u16)
        n287 = Greater?(x=w604, y=w603) -> (0:w601:bool)
        n288 = Select(t=Aquire_State."AlignWave" ("Acquire State"), s=w601, f=Aquire_State."Idle") -> (s? t:f=w609:T3)
        n289 = xnode ("FIFO Method Node")("Element"=w601, "Timeout"=0) -> ()  [unwired: 1 in, 2 out]
      }
    }
  }
  n290 = while "Configuration Loop" {
    stop <- FALSE stop-if-true
    # "After the NI 5772 is powered on, the CLIP core provides the module with a default configuration. This loop updates the host VI to the status of the NI 5772 through the Initalization Done Signal. Additionally, this loop configures the Sample clock selection for the NI 5772. Refer to the Clock Select (Host).vi Host VI for more information about how this example configures the clock."
    n291 = xnode "FPGA I/O Node"("IO Module\\User Command"="User Command", "IO Module\\User Data 0"="User Data 0", "IO Module\\User Data 1"="User Data 1", "IO Module\\User Command Commit"="User Command Commit") -> ("IO Module\\User Command Idle"=→"User Command Idle":bool, "IO Module\\User Command Status"=→"User Command Status":u8, "IO Module\\PLL Locked"=→"PLL Locked":bool, "IO Module\\User Error"=w619:u8, "IO Module\\Initialization Done"=→"Configured?":bool)  [unwired: 9 in, 9 out]
    n292 = Not Equal To 0?(x=w619) -> (x != 0?=→"User Error":bool)
  }
  n293 = while "Data Validation/Calculation Loop" {
    stop <- FALSE stop-if-true
    n294 = Scale By Power Of 2(n="AvgCount_powerOf2", x=1 ("Timeout")) -> (x*2^n=w645:i32)
    n295 = To Unsigned Word Integer(number=w645) -> (unsigned 16bit integer=w642:u16)
    n296 = Multiply(x="Delay (us)", y=sgl 200.0) -> (x*y=w638:u16)
    n297 = Divide(x="WaveSampleCount", y="Wave Sampling Rate") -> (x/y=w629:sgl)
    n298 = In Range and Coerce(upper limit=u16 65535, x=w638, lower limit=u16 1) -> (coerced(x)=w630:u16)  [unwired: 1 out]
    "Delay after Trig [cycles]" <- w630
    n299 = In Range and Coerce(upper limit=u16 65535, x=w642, lower limit=u16 1) -> (coerced(x)=→"AvgCount":u16)  [unwired: 1 out]
    n300 = Multiply(x=w629, y=sgl 200000000.0) -> (x*y=w626:sgl)
    n301 = Add(x="Samples Per Trigger", y=w630) -> (x+y=w627:u16)
    n302 = Subtract(x=w626, y=w627) -> (x-y=→"WaitForWave\nCompletion":u16)
    n303 = call "Loop Timer"("Count(uSec)"=u32 100 ("Count(mSec)")) -> ()  [unwired: 1 out]
  }
  n304 = while "TrigOut Loop" {
    stop <- FALSE stop-if-true
    n305 = xnode ("FIFO Method Node")("Timeout"=0) -> ("Element"=w648:bool)  [unwired: 1 in, 2 out]
    n306 = case shown="True" w648 {
      frame False {
      }
      frame True {
        n307 = flat-sequence {
          frame #0 {
            n308 = xnode "FPGA I/O Node"("PXI_Trig1"=TRUE) -> ()  [unwired: 1 in, 1 out]
          }
          frame #1 {
            n309 = call "Wait"("Count(Ticks)"=u32 20 ("Count(uSec)")) -> ()  [unwired: 1 out]
          }
          frame #2 {
            n310 = xnode "FPGA I/O Node"("PXI_Trig1"=FALSE) -> ()  [unwired: 1 in, 1 out]
          }
        }
      }
    }
  }
  n311 = node-c288() -> (w11:T4)  [unwired: 1 in]
  n312 = timed-loop "Trigger In Loop" {
    timing: w11 -> [_]
    timing-out: [_] -> w10
    stop <- FALSE stop-if-true
    # "Triggering is handeled in the 40MHz Loop to remove the signal Jitter and false triggers"
    n313 = xnode "FPGA I/O Node"() -> ("IO Module\\Asynchronous Trigger Input"=w659:bool)  [unwired: 1 in, 1 out]
    n314 = call <instrlib>:"Detect Rising Edge.vi"("signal"=w659) -> ("edge detected"=w656:bool)  [unwired: 14 in]
    n315 = xnode ("FIFO Method Node")("Element"=w659, "Timeout"=0) -> ()  [unwired: 1 in, 2 out]
    n316 = call-poly <instrlib>:"Count Up.vi"("increment"=w656, "reset"="Clear Count") -> ("count out"=→"Trig Count":u64)  [unwired: 13 in]
  }
  n317 = node-c288(w10) -> ()
  n318 = node-c288(w6) -> ()
  n319 = node-c288(w15) -> ()
